vi "Destruct Messenger.vi"(8 "error in (no error)":errorcluster, 11 "Queue Messenger Composite in":refnum<class "Tree-ArrayLocation Queue Messenger.lvclass">) -> (0 "error out":errorcluster, 3 "Queue Messenger Composite out":refnum<class "Tree-ArrayLocation Queue Messenger.lvclass">)   [LabVIEW 2019, in "Tree-ArrayLocation Queue Messenger.lvclass"]
uses:
  Tree-ArrayLocation Queue Messenger.lvclass
  Tree-ArrayLocation Queue Messenger.lvclass/Tree-ArrayLocation Queue Messenger.ctl
  Ancestor Class/Messenger/Messenger Composite/Messenger Composite.lvclass
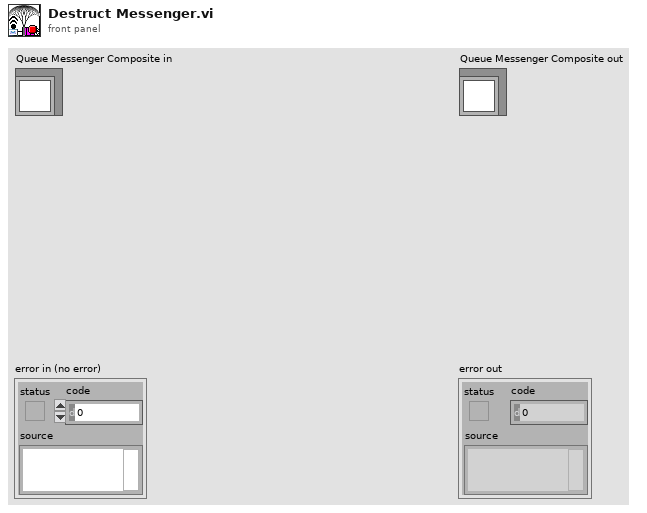
[diagram p1: front panel]
types:
  T1 = typedef "Message Queue.ctl" = refnum<queue>
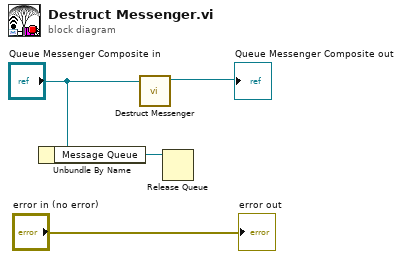
[diagram p0: block diagram]
diagram:
  n1 = Unbundle By Name("Queue Messenger Composite in") -> ("Message Queue"=w3:T1)
  n2 = call-parent "Destruct Messenger.vi"("Messenger Component in"="Queue Messenger Composite in") -> ("Messenger Component out"=→"Queue Messenger Composite out":refnum<class "Tree-ArrayLocation Queue Messenger.lvclass">)  [unwired: 9 in, 1 out]
  n3 = Release Queue(queue=w3) -> ()  [unwired: 2 in, 3 out]
  "error out" <- "error in (no error)"
